vi "EOL CAN_Get_Motor_Voltage.vi"(11 "NetworkObjHandle":T1) -> (1 "Motor Voltage":dbl, 2 "TxRx Data":string[][](array[string]), 3 "Response Good?":bool)   [LabVIEW 2018]
uses:
  <vilib>/nican/nican.llb/xobjhandle.ctl
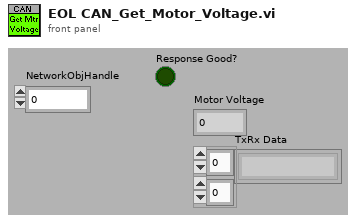
[diagram p1: front panel]
types:
  T1 = typedef "xobjhandle.ctl" = u32
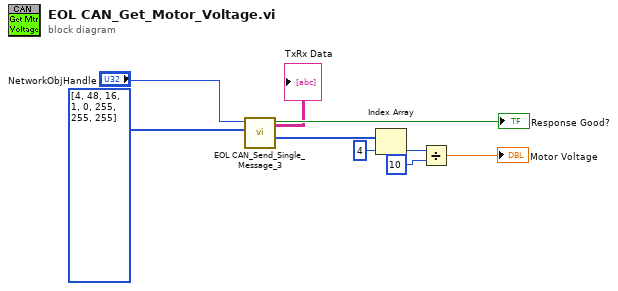
[diagram p0: block diagram]
diagram:
  n1 = call <userlib>:"EOL CAN_Send_Single_Message_3.vi"("Tx Msg"=u8[] [4, 48, 16, 1, 0, 255, 255, 255] ("Transmit Data"), "NetworkObjHandle"="NetworkObjHandle") -> ("Rx Message"=w4:u8[], "Response Good?"=→"Response Good?":bool, "TxRx Data"=→"TxRx Data":string[][])  [unwired: 6 in, 1 out]
  n2 = Index Array(array=w4, index=4) -> (element=w6:u8)
  n3 = Divide(x=w6, y=u8 10) -> (x/y=→"Motor Voltage":dbl)
